vi "Next_Filepath(SubVI).vi"(8 "error in (no error)":errorcluster, 11 "Input filepath":path) -> (0 "error out":errorcluster, 3 "Next  filepath":path)   [LabVIEW 2014]
doc: "SubVI increase filename and construct new filepath for open nex data"
panel:
  out "NEW string":string
  out "name1":string
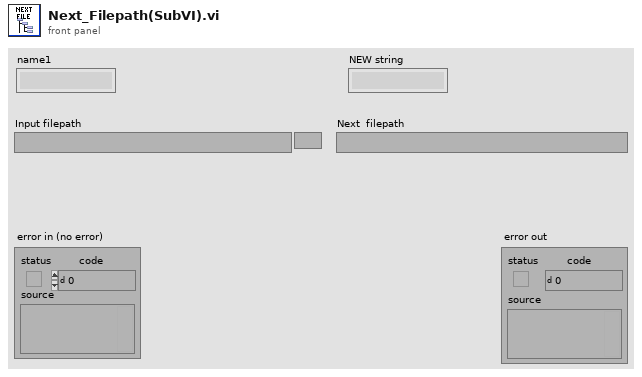
[diagram p1: front panel]
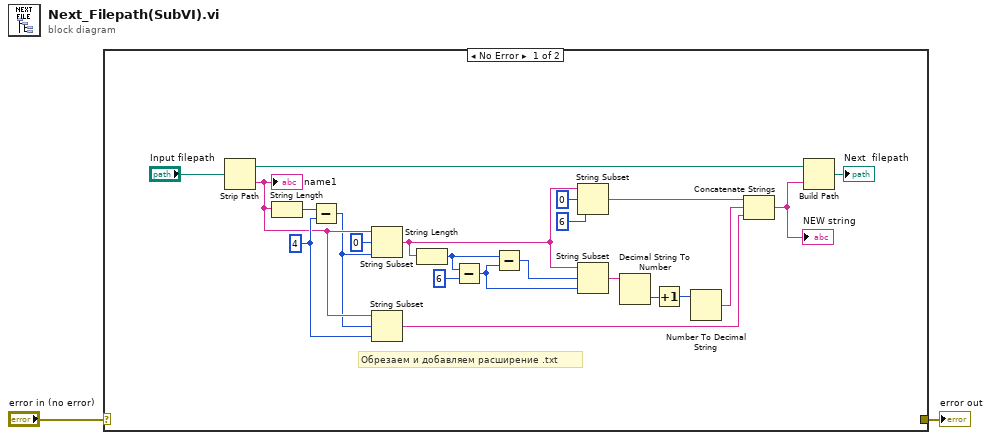
[diagram p0: block diagram]
diagram:
  n1 = case shown="No Error" "error in (no error)" {
    selector: "error in (no error)" -> [_ w25]
    tunnel: [_ w25] -> w1
    frame No Error {
      w19 = 4 ("y")
      # "Обрезаем и добавляем расширение .txt"
      n2 = Strip Path(path="Input filepath") -> (stripped path=w21:path, name=w18:string)
      "name1" <- w18
      n3 = String Length(string=w18) -> (length=w7:i32)
      n4 = Subtract(x=w7, y=w19) -> (x-y=w17:i32)
      n5 = String Subset(string=w18, offset (0)=0, length (rest)=w17) -> (substring=w11:string)
      n6 = String Subset(string=w18, offset (0)=w17, length (rest)=w19) -> (substring=w20:string)
      n7 = String Length(string=w11) -> (length=w5:i32)
      n8 = Subtract(x=w5, y=6) -> (x-y=w3:i32)
      n9 = Subtract(x=w5, y=w3) -> (x-y=w4:i32)
      n10 = String Subset(string=w11, offset (0)=0, length (rest)=6 ("length (rest)")) -> (substring=w15:string)
      n11 = String Subset(string=w11, offset (0)=w4, length (rest)=w3) -> (substring=w10:string)
      n12 = Decimal String To Number(string=w10) -> (number=w13:i32)  [unwired: 2 in, 1 out]
      n13 = Increment(x=w13) -> (x+1=w14:i32)
      n14 = Number To Decimal String(number=w14) -> (decimal integer string=w16:string)  [unwired: 1 in]
      n15 = Concatenate Strings(w15, w16, w20) -> (w22:string)
      "NEW string" <- w22
      n16 = Build Path(base path=w21, name or relative path=w22) -> (appended path=→"Next  filepath":path)
    }
    frame Error {
    }
  }
  "error out" <- w1
